vi "Build All.vi"(10 "Changes":string, 11 "Version Increment":T2) -> (1 "Build Error":bool, 2 "Status":string, 3 "Version":T1, 5 "Description":string)   [LabVIEW 2021]
uses:
  <vilib>/CIF Foundation/CIF LabVIEW Scripting/LV Scripting/Typedef/Version Increment.ctl
  <vilib>/CIF Foundation/CIF LabVIEW Scripting/LV Scripting/Typedef/Version.ctl
  <vilib>/CIF Foundation/CIF Core/CIFUtilities/Scripting/Build Libraries/LabVIEW Build Script/LabVIEW Build Script.lvclass/LabVIEW Build Script.ctl
  <vilib>/CIF Foundation/CIF LabVIEW Scripting/LV Scripting/SubVIs/Add Scripting Error.vi
  <vilib>/CIF Foundation/CIF Utilities/Errors/Append Error Location.vi
  <vilib>/AppBuilder/AB_API_Simple/Build (path).vi
  <vilib>/AppBuilder/AB_API_Simple/NI_App_Builder_API.lvlib
  <vilib>/CIF Foundation/CIF LabVIEW Scripting/LV Scripting/LV Scripting Utilities.lvlib
  <vilib>/CIF Foundation/CIF Core/CIFUtilities/Scripting/Build Libraries/LabVIEW Build Script/LabVIEW Build Script.lvclass
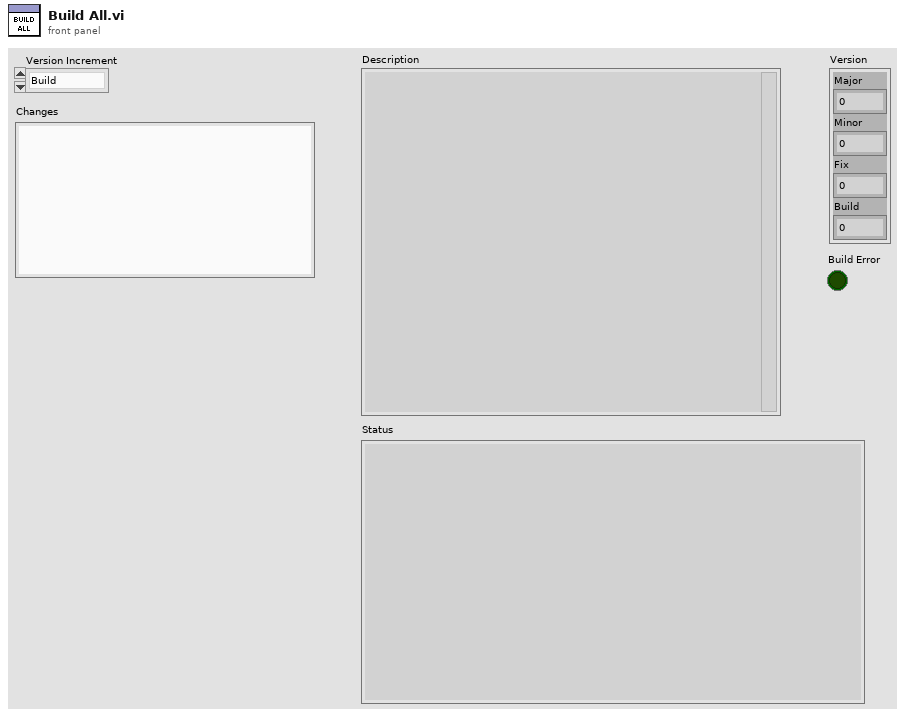
[diagram p1: front panel]
types:
  T1 = typedef "Version.ctl" = cluster{"Major":u16, "Minor":u16, "Fix":u16, "Build":u16}
  T2 = typedef "LV Scripting Utilities.lvlib/Version Increment.ctl" = enum16{"Build", "Fix", "Minor", "Major"}
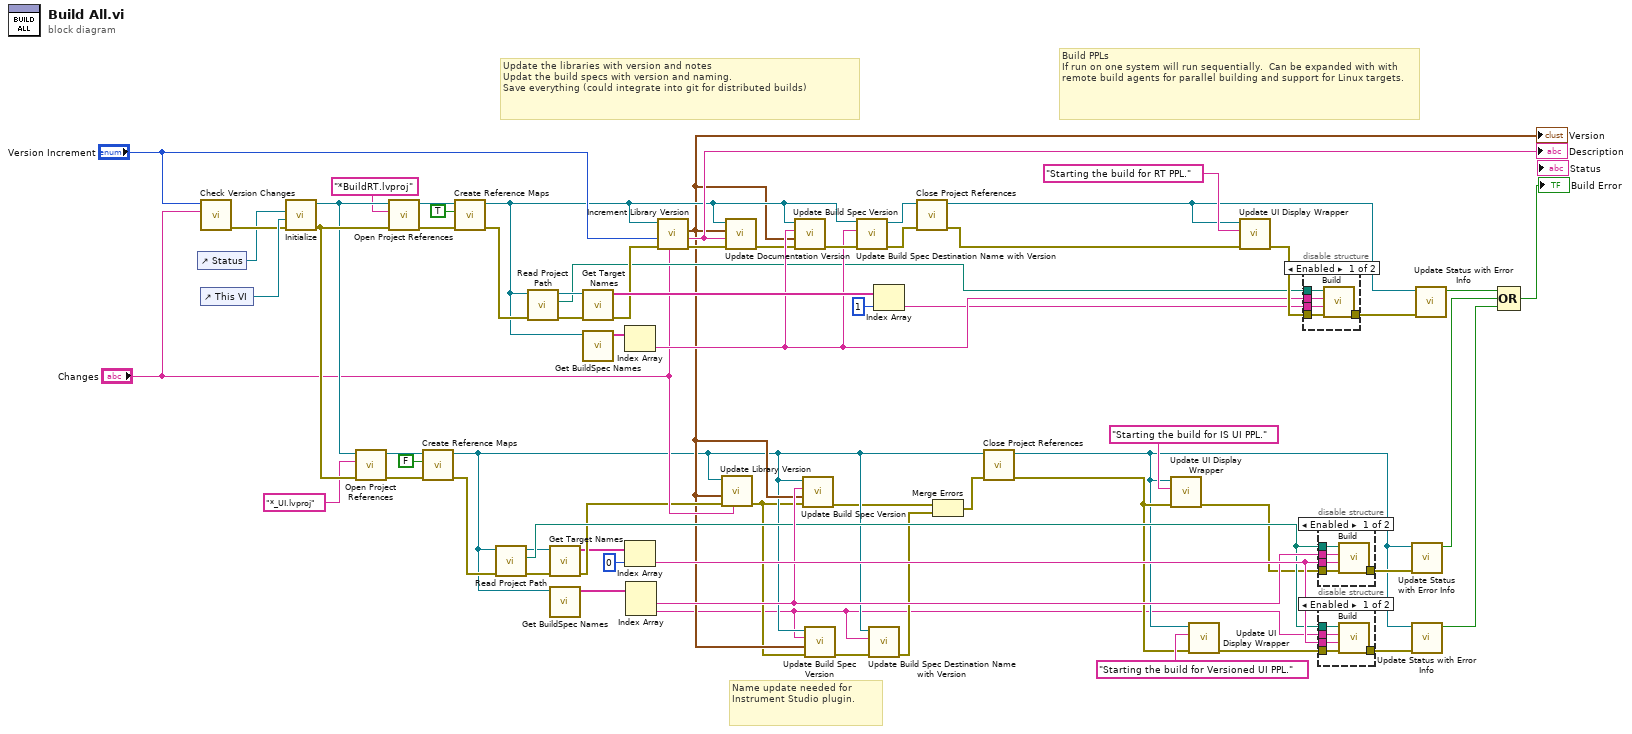
[diagram p0: block diagram]
diagram:
  # "Name update needed for Instrument Studio plugin."
  # "Build PPLs\nIf run on one system will run sequentially.  Can be expanded with with remote build agents for parallel building and support for Linux targets."
  # "Update the libraries with version and notes\nUpdat the build specs with version and naming.\nSave everything (could integrate into git for distributed builds)"
  n1 = control-ref of="Status"() -> (w47:refnum<vi>)
  n2 = call <vilib>:"Check Version Changes.vi"("Changes"="Changes", "Version Increment"="Version Increment") -> ("error out"=w52:errorcluster)  [unwired: 9 in]
  n3 = control-ref of="This VI"() -> (w56:refnum<vi>)
  n4 = call <vilib>:"Initialize.vi"("error in (no error)"=w52, "Calling VI"=w56, "UI Display"=w47) -> ("error out"=w67:errorcluster, "LabVIEW Build Script out"=w66:refnum<class "LabVIEW Build Script.lvclass">)  [unwired: 7 in]
  n5 = call <vilib>:"Open Project References.vi"("error in (no error)"=w67, "Search Pattern"="*_UI.lvproj" ("pattern"), "LabVIEW Build Script in"=w66) -> ("error out"=w22:errorcluster, "LabVIEW Build Script out"=w21:refnum<class "LabVIEW Build Script.lvclass">)  [unwired: 7 in]
  n6 = call <vilib>:"Open Project References.vi"("error in (no error)"=w67, "Search Pattern"="*BuildRT.lvproj" ("pattern"), "LabVIEW Build Script in"=w66) -> ("error out"=w50:errorcluster, "LabVIEW Build Script out"=w49:refnum<class "LabVIEW Build Script.lvclass">)  [unwired: 7 in]
  n7 = call <vilib>:"Create Reference Maps.vi"("error in (no error)"=w22, "RT Target"=FALSE, "LabVIEW Build Script in"=w21) -> ("error out"=w14:errorcluster, "LabVIEW Build Script out"=w6:refnum<class "LabVIEW Build Script.lvclass">)  [unwired: 7 in]
  n8 = call <vilib>:"Create Reference Maps.vi"("error in (no error)"=w50, "RT Target"=TRUE, "LabVIEW Build Script in"=w49) -> ("error out"=w61:errorcluster, "LabVIEW Build Script out"=w33:refnum<class "LabVIEW Build Script.lvclass">)  [unwired: 7 in]
  n9 = call <vilib>:"Read Project Path.vi"("error in (no error)"=w14, "LabVIEW Build Script in"=w6) -> ("error out"=w13:errorcluster, "Project Path"=w28:path, "LabVIEW Build Script out"=w12:refnum<class "LabVIEW Build Script.lvclass">)  [unwired: 7 in]
  n10 = call <vilib>:"Read Project Path.vi"("error in (no error)"=w61, "LabVIEW Build Script in"=w33) -> ("error out"=w62:errorcluster, "Project Path"=w43:path, "LabVIEW Build Script out"=w63:refnum<class "LabVIEW Build Script.lvclass">)  [unwired: 7 in]
  n11 = call <vilib>:"Get Target Names.vi"("error in (no error)"=w13, "LabVIEW Build Script in"=w12) -> ("error out"=w18:errorcluster, "Project Targets"=w16:string[])  [unwired: 8 in]
  n12 = call <vilib>:"Get BuildSpec Names.vi"("LabVIEW Build Script in"=w6) -> ("BuildSpecs"=w17:string[])  [unwired: 10 in]
  n13 = call <vilib>:"Get Target Names.vi"("error in (no error)"=w62, "LabVIEW Build Script in"=w63) -> ("error out"=w57:errorcluster, "Project Targets"=w59:string[])  [unwired: 8 in]
  n14 = call <vilib>:"Get BuildSpec Names.vi"("LabVIEW Build Script in"=w33) -> ("BuildSpecs"=w58:string[])  [unwired: 10 in]
  n15 = Index Array(array=w58) -> (element=w45:string)  [unwired: 1 in]
  n16 = Index Array(array=w16, index=0) -> (element=w30:string)
  n17 = Index Array(array=w17) -> (element #1=w29:string, element #2=w1:string)  [unwired: 2 in]
  n18 = call <vilib>:"Increment Library Version.vi"("Changes"="Changes", "error in (no error)"=w57, "Version Increment"="Version Increment", "LabVIEW Build Script in"=w33) -> ("error out"=w40:errorcluster, "Description"=w38:string, "Version"=w7:T1)  [unwired: 5 in]
  "Description" <- w38
  "Version" <- w7
  n19 = call <vilib>:"Update Library Version.vi"("Changes"="Changes", "error in (no error)"=w18, "Version"=w7, "LabVIEW Build Script in"=w6) -> ("error out"=w2:errorcluster)  [unwired: 6 in, 1 out]
  n20 = call <vilib>:"Update Documentation Version.vi"("error in (no error)"=w40, "Description"=w38, "Version"=w7, "LabVIEW Build Script in"=w33) -> ("error out"=w39:errorcluster)  [unwired: 7 in]
  n21 = call <vilib>:"Update Build Spec Version.vi"("error in (no error)"=w39, "Version"=w7, "Search Pattern"=w45, "LabVIEW Build Script in"=w33) -> ("error out"=w53:errorcluster)  [unwired: 7 in]
  n22 = call <vilib>:"Update Build Spec Version.vi"("error in (no error)"=w2, "Version"=w7, "Search Pattern"=w29, "LabVIEW Build Script in"=w6) -> ("error out"=w5:errorcluster)  [unwired: 7 in]
  n23 = call <vilib>:"Update Build Spec Version.vi"("error in (no error)"=w2, "Version"=w7, "Search Pattern"=w1, "LabVIEW Build Script in"=w6) -> ("error out"=w23:errorcluster)  [unwired: 7 in]
  n24 = call <vilib>:"Update Build Spec Destination Name with Version.vi"("error in (no error)"=w53, "Search Pattern"=w45, "LabVIEW Build Script in"=w33) -> ("error out"=w55:errorcluster, "LabVIEW Build Script out"=w54:refnum<class "LabVIEW Build Script.lvclass">)  [unwired: 7 in]
  n25 = call <vilib>:"Update Build Spec Destination Name with Version.vi"("error in (no error)"=w23, "Search Pattern"=w1, "LabVIEW Build Script in"=w6) -> ("error out"=w4:errorcluster)  [unwired: 7 in, 1 out]
  n26 = Index Array(array=w59, index=1) -> (element=w44:string)
  n27 = call <vilib>:"Close Project References.vi"("error in (no error)"=w55, "LabVIEW Build Script in"=w54) -> ("error out"=w64:errorcluster, "LabVIEW Build Script out"=w35:refnum<class "LabVIEW Build Script.lvclass">)  [unwired: 8 in]
  n28 = Merge Errors(w5, w4) -> (w3:errorcluster)
  n29 = call <vilib>:"Close Project References.vi"("error in (no error)"=w3, "LabVIEW Build Script in"=w6) -> ("error out"=w25:errorcluster, "LabVIEW Build Script out"=w8:refnum<class "LabVIEW Build Script.lvclass">)  [unwired: 8 in]
  n30 = call <vilib>:"Update UI Display Wrapper.vi"("error in (no error)"=w25, "Update for Display"="Starting the build for IS UI PPL.", "LabVIEW Build Script in"=w8) -> ("error out"=w20:errorcluster)  [unwired: 8 in]
  n31 = call <vilib>:"Update UI Display Wrapper.vi"("error in (no error)"=w25, "Update for Display"="Starting the build for Versioned UI PPL.", "LabVIEW Build Script in"=w8) -> ("error out"=w27:errorcluster)  [unwired: 8 in]
  n32 = call <vilib>:"Update UI Display Wrapper.vi"("error in (no error)"=w64, "Update for Display"="Starting the build for RT PPL.", "LabVIEW Build Script in"=w35) -> ("error out"=w46:errorcluster)  [unwired: 8 in]
  n33 = disable-structure shown="Enabled" {
    disable-tunnel: w43 -> [w72 _]
    disable-tunnel: w44 -> [w71 _]
    disable-tunnel: w45 -> [w70 _]
    disable-tunnel: w46 -> [w69 w73]
    disable-tunnel: [w68 w73] -> w36
    frame Enabled {
      n34 = call-poly <vilib>:"Build.vi"("error in (no error)"=w69, "Name of target (My Computer)"=w71, "Name of build specification (if empty: build all)"=w70, "Path to project"=w72) -> ("error out"=w68:errorcluster)  [unwired: 6 in, 1 out]
    }
    frame Disabled {
    }
  }
  n35 = disable-structure shown="Enabled" {
    disable-tunnel: w28 -> [w78 _]
    disable-tunnel: w30 -> [w77 _]
    disable-tunnel: w29 -> [w76 _]
    disable-tunnel: w20 -> [w75 w79]
    disable-tunnel: [w74 w79] -> w10
    frame Enabled {
      n36 = call-poly <vilib>:"Build.vi"("error in (no error)"=w75, "Name of target (My Computer)"=w77, "Name of build specification (if empty: build all)"=w76, "Path to project"=w78) -> ("error out"=w74:errorcluster)  [unwired: 6 in, 1 out]
    }
    frame Disabled {
    }
  }
  n37 = disable-structure shown="Enabled" {
    disable-tunnel: w28 -> [w84 _]
    disable-tunnel: w30 -> [w83 _]
    disable-tunnel: w1 -> [w82 _]
    disable-tunnel: w27 -> [w81 w85]
    disable-tunnel: [w80 w85] -> w9
    frame Enabled {
      n38 = call-poly <vilib>:"Build.vi"("error in (no error)"=w81, "Name of target (My Computer)"=w83, "Name of build specification (if empty: build all)"=w82, "Path to project"=w84) -> ("error out"=w80:errorcluster)  [unwired: 6 in, 1 out]
    }
    frame Disabled {
    }
  }
  n39 = call <vilib>:"Update Status with Error Info.vi"("error in (no error)"=w10, "LabVIEW Build Script"=w8) -> ("Error"=w32:bool)  [unwired: 9 in]
  n40 = call <vilib>:"Update Status with Error Info.vi"("error in (no error)"=w9, "LabVIEW Build Script"=w8) -> ("Error"=w31:bool)  [unwired: 9 in]
  n41 = call <vilib>:"Update Status with Error Info.vi"("error in (no error)"=w36, "LabVIEW Build Script"=w35) -> ("Error"=w34:bool)  [unwired: 9 in]
  n42 = Compound Arithmetic op=OR(w34, w32, w31) -> (→"Build Error":bool)
